vi "Lidar Encoder Reader.vi"   [LabVIEW 2010]
uses:
  <vilib>/eio/EIONode/EIONode.xnode
  Motor Encoder Global.vi
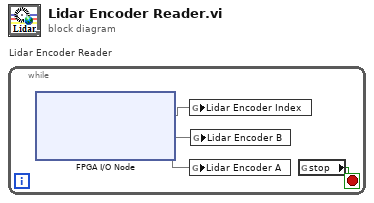
[diagram p0: block diagram]
diagram:
  n1 = while "Lidar Encoder Reader" {
    stop <- w1 stop-if-true
    n2 = xnode "FPGA I/O Node"() -> ("Lidar Encoder Index"=w4, "Lidar Encoder B"=w3, "Lidar Encoder A"=w2)  [unwired: 3 in, 3 out]
    n3 = global write "Motor Encoder Global.vi" "Lidar Encoder Index"(w4) -> ()
    n4 = global write "Motor Encoder Global.vi" "Lidar Encoder A"(w2) -> ()
    n5 = global write "Motor Encoder Global.vi" "Lidar Encoder B"(w3) -> ()
    n6 = global read "Motor Encoder Global.vi" "stop"() -> (w1:bool)
  }
